vi "Interpolate 2 Arrays.vi"(1 "Y2":dbl, 2 "Z":dbl, 3 "Y1":dbl) -> (0 "Yi":dbl)   [LabVIEW 2020]
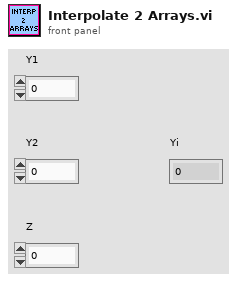
[diagram p1: front panel]
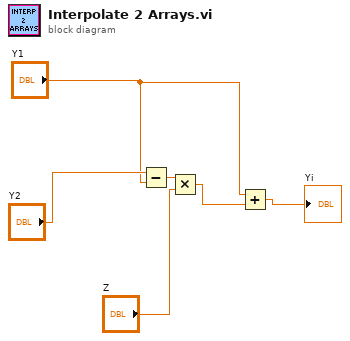
[diagram p0: block diagram]
diagram:
  n1 = Subtract(x="Y2", y="Y1") -> (x-y=w5:dbl)
  n2 = Multiply(x=w5, y="Z") -> (x*y=w2:dbl)
  n3 = Add(x="Y1", y=w2) -> (x+y=→"Yi":dbl)
